vi "Traffic Light.vi"() -> ()   [LabVIEW 2013]
doc: "This VI is a simulation of traffic light.\nWere the traffic light controller provides for red,yellow and green light for every direction-\n-North Bound\n-South Bound\n-East Bound\n-West Bound\nAnd the second red, yellow and green list are provided for the left hand turn lane-\n-North Bound Left\n-South Bound Left\n-East Bound Left\n-West Bound Left\n\nThe period of time that light will be on is\n-Red: 4 sec\n-Yellow: 2 sec\n-Greeen: 4 sec\n\nThe left turn sequence eill be ON only when there will be the vehicle on the sensor."
uses:
  Controls/Traffic light.ctl
  Controls/Traffic_light_left.ctl
  Controls/States.ctl
  Controls/Sensor.ctl
panel:
  out "Enum":T1
  in  "North  Sensor":bool
  in  "Start":bool caption="stop"
  out "South Bound Left":T2
  out "South Bound":T3={"R"=TRUE, "Y"=FALSE, "G"=FALSE}
  out "West Bound Left":T2
  out "West Bound":T3={"R"=TRUE, "Y"=FALSE, "G"=FALSE}
  out "East Bound Left":T2
  out "East Bound":T3={"R"=TRUE, "Y"=FALSE, "G"=FALSE}
  in  "stop":bool
  in  "West Sensor":bool
  in  "East Sensor":bool
  in  "South Sensor":bool
  out "North Bound Left":T2
  out "North Bound":T3={"R"=TRUE, "Y"=FALSE, "G"=FALSE}
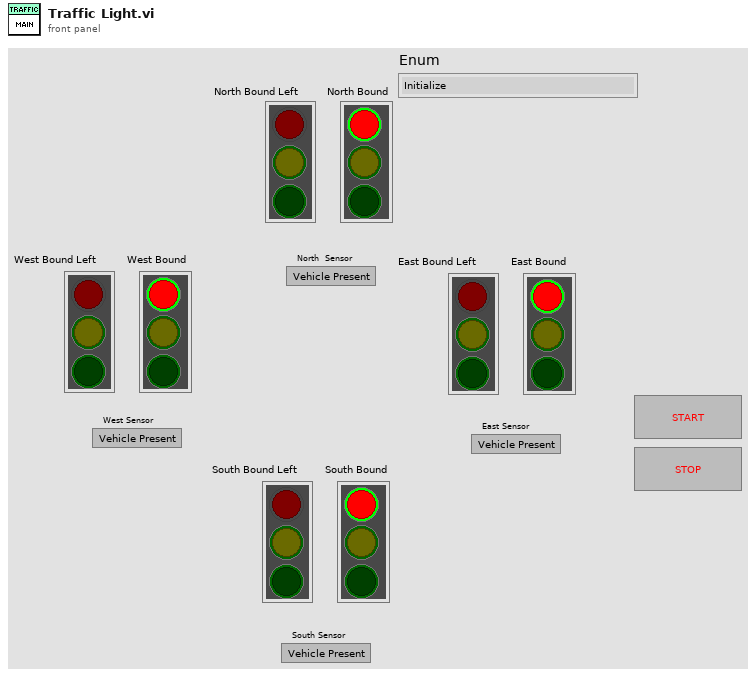
[diagram p1: front panel]
types:
  T1 = typedef "States.ctl" = enum16{"Initialize", "NS Green", "NS Yellow", "EW Green", "EW Yellow", "NS Left Green", "NS Left Yellow", "EW Left Green", "EW Left Yellow", "Stop"}
  T2 = typedef "Traffic_light_left.ctl" = cluster{"R":bool, "Y":bool, "G":bool}
  T3 = typedef "Traffic light.ctl" = cluster{"R":bool, "Y":bool, "G":bool}
  T4 = cluster{"North Bound":T3, "South Bound":T3, "East Bound":T3, "West Bound":T3, "North Bound Left":T2, "South Bound Left":T2, "East Bound Left":T2, "West Bound Left":T2}
  T5 = typedef "Sensor.ctl" = enum16{"Get", "Set"}
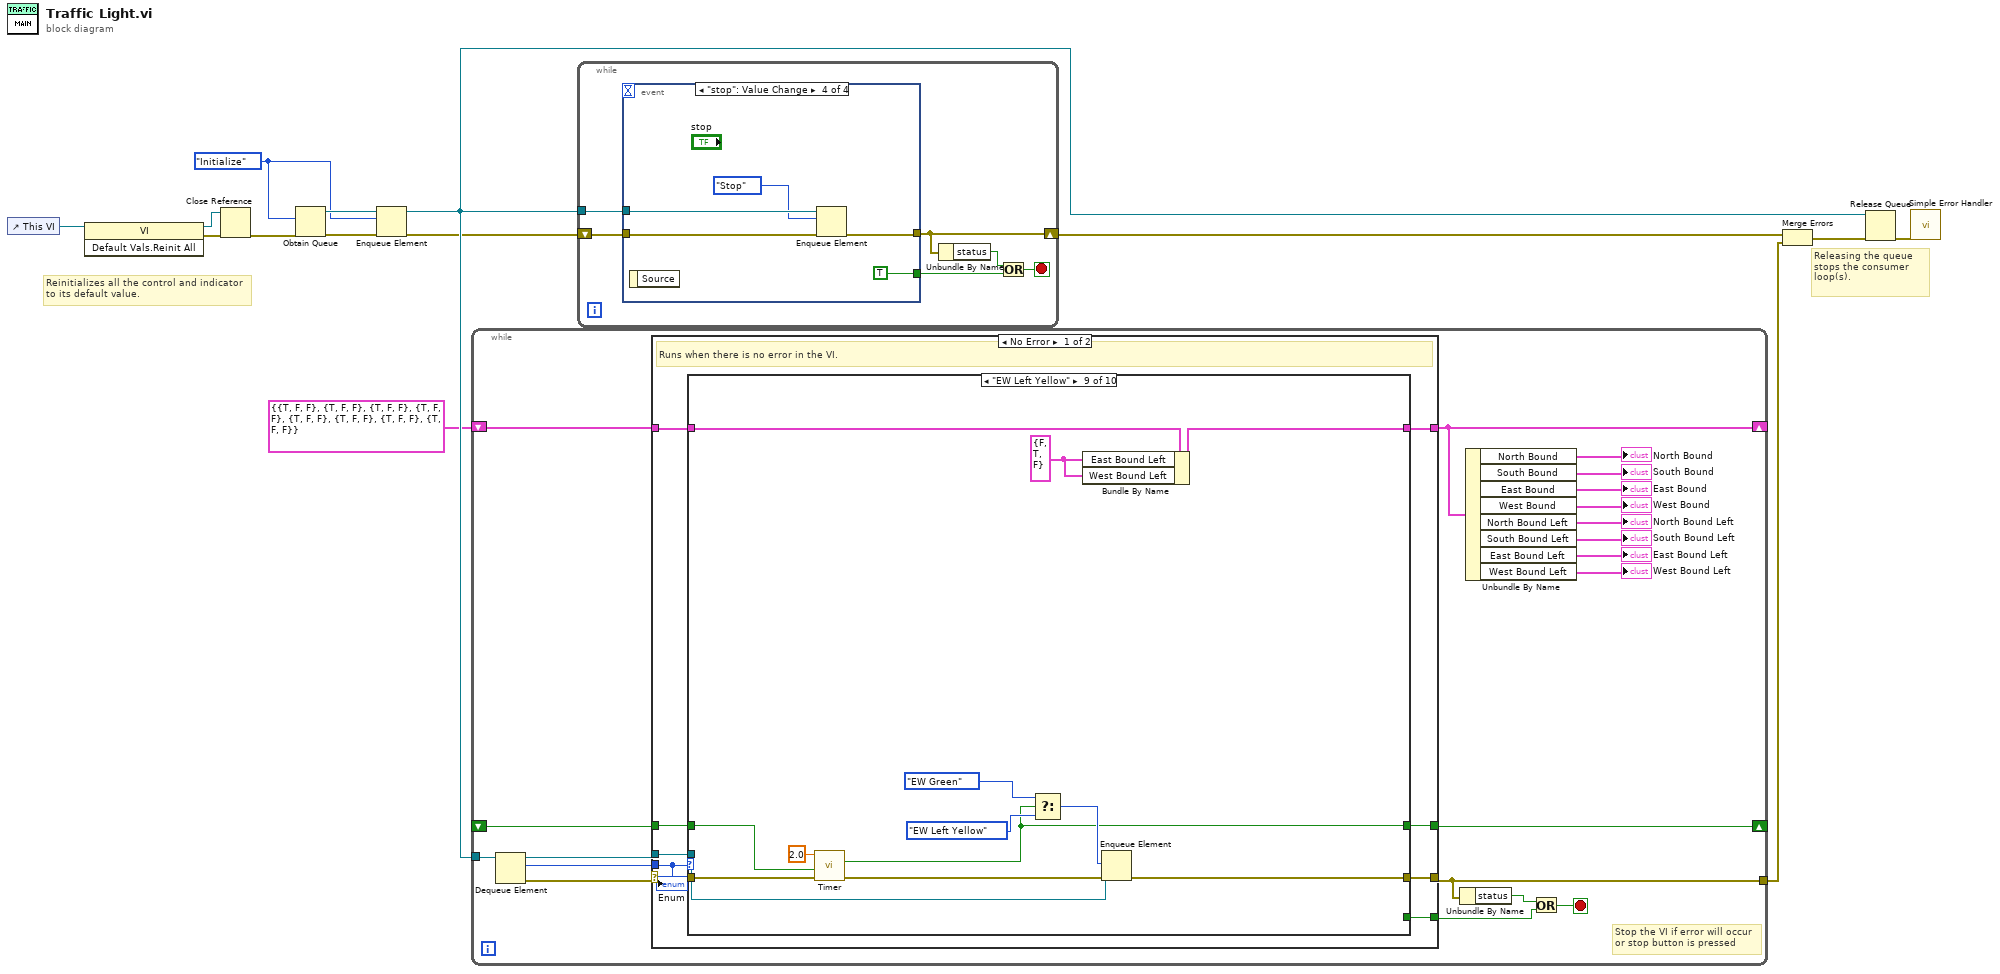
[diagram p0: block diagram]
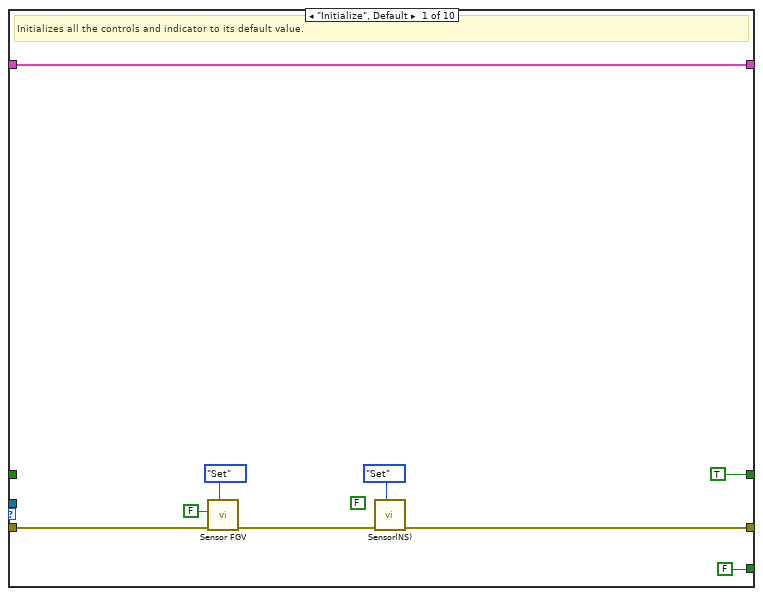
[diagram p2: hidden frame]
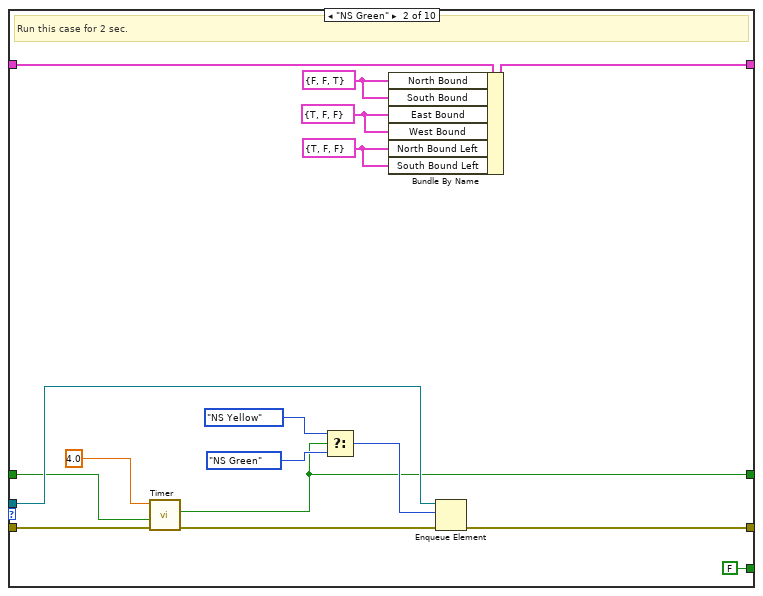
[diagram p3: hidden frame]
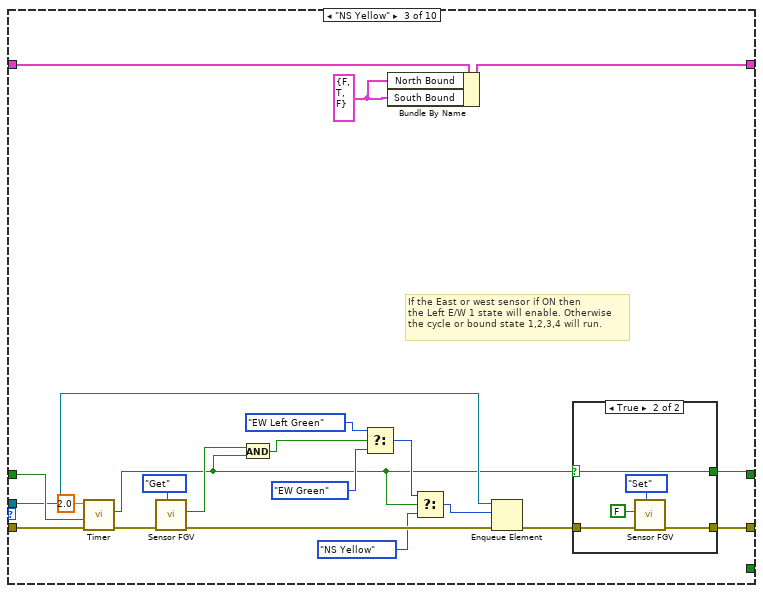
[diagram p4: hidden frame]
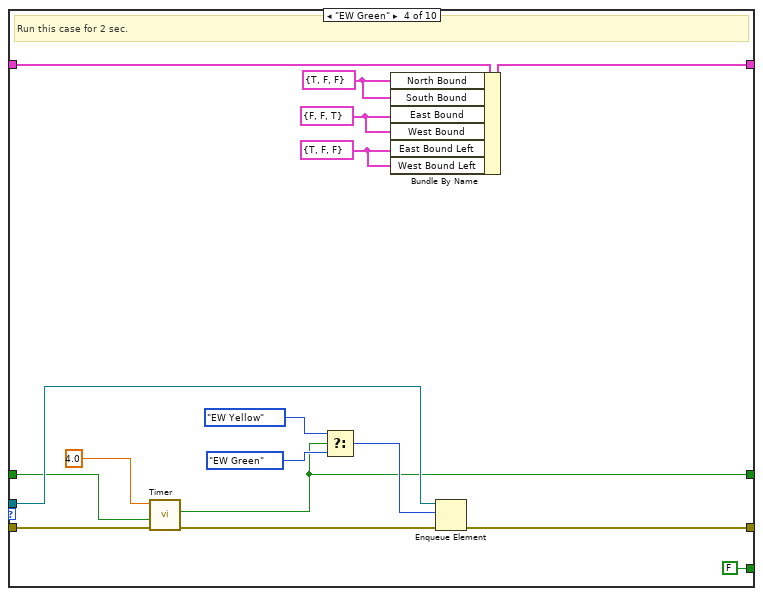
[diagram p6: hidden frame]
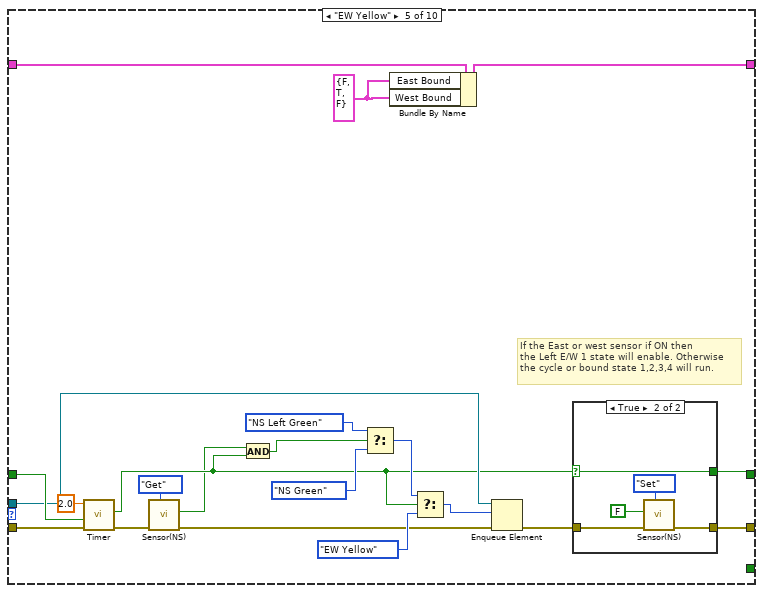
[diagram p7: hidden frame]
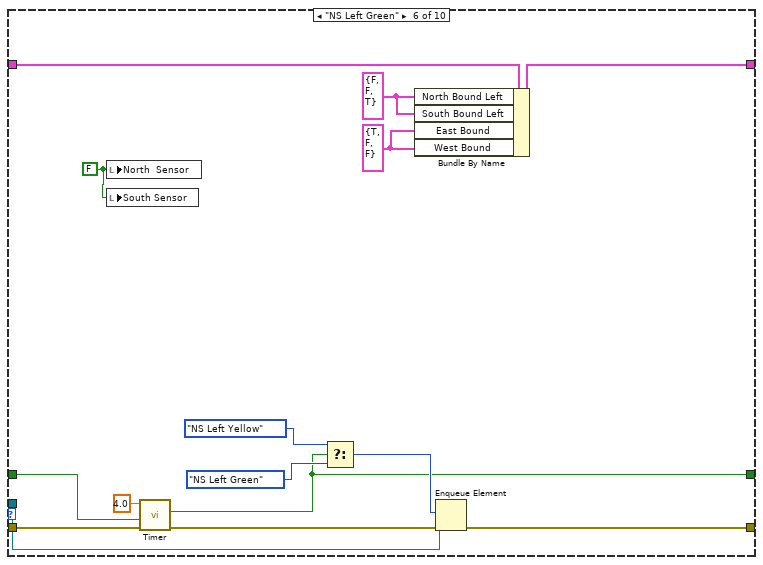
[diagram p9: hidden frame]
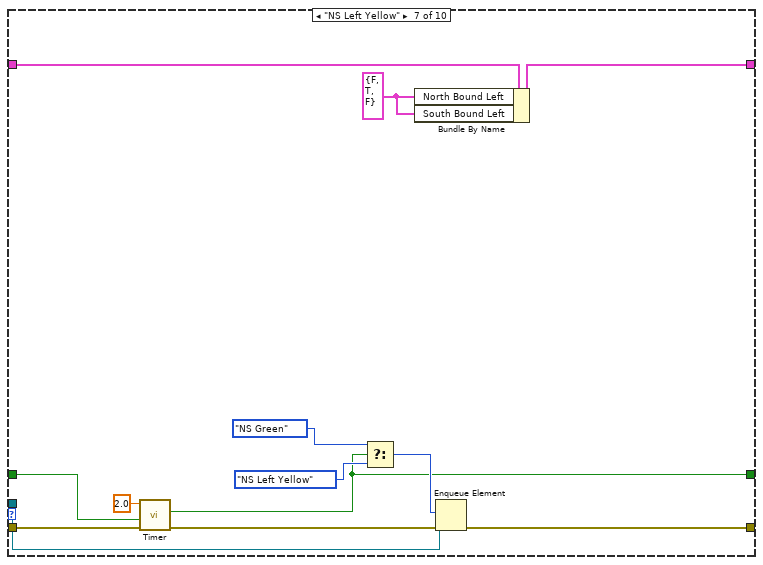
[diagram p10: hidden frame]
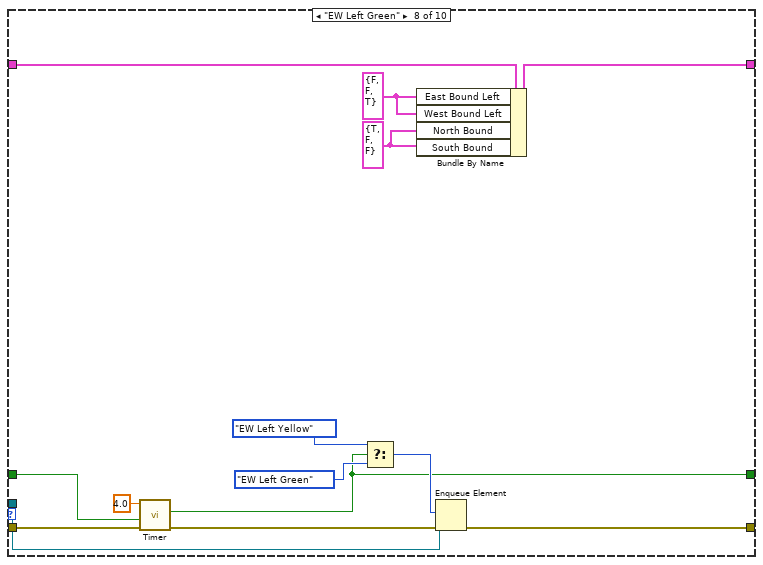
[diagram p11: hidden frame]
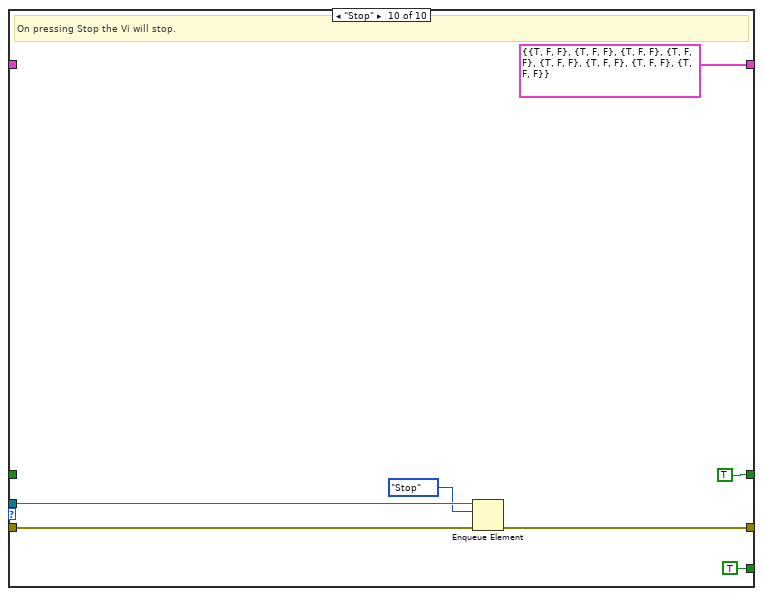
[diagram p12: hidden frame]
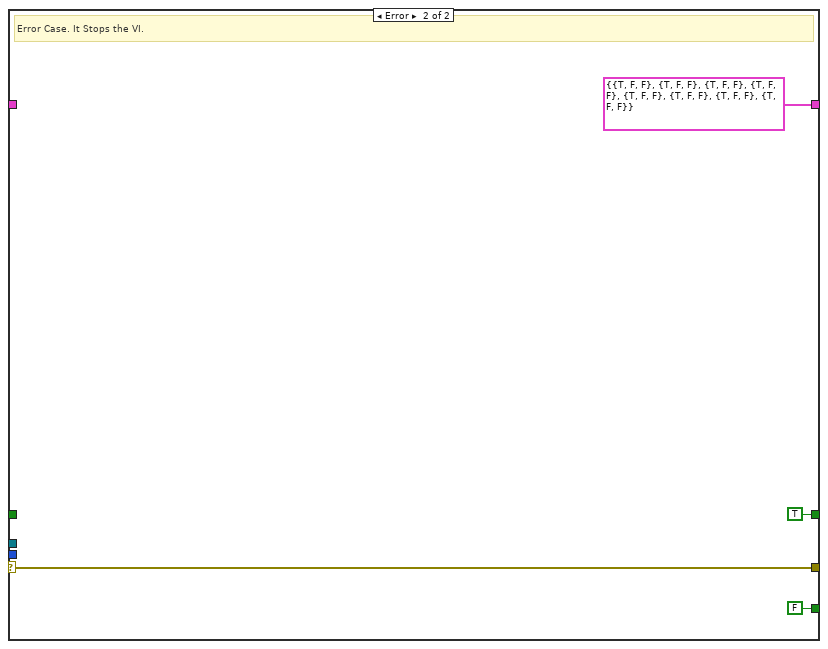
[diagram p13: hidden frame]
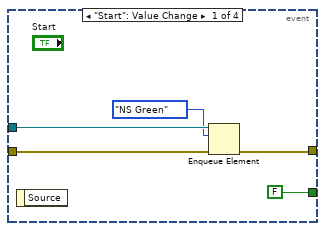
[diagram p14: hidden frame]
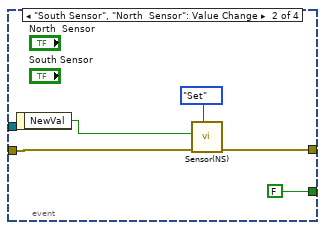
[diagram p15: hidden frame]
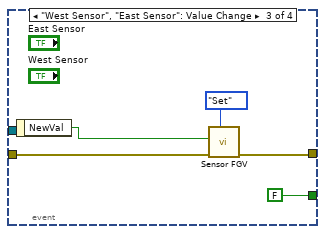
[diagram p16: hidden frame]
diagram:
  w10 = States."Initialize"
  # "Reinitializes all the control and indicator\nto its default value."
  # "Releasing the queue stops the consumer loop(s)."
  n1 = control-ref of="This VI"() -> (w9:refnum<vi>)
  n2 = invoke class="VI" method="Default Vals.Reinit All"(reference=w9) -> (reference out=w7:refnum<vi>, error out=w8:errorcluster)  [unwired: 2 in, 1 out]
  n3 = Close Reference(reference=w7, error in (no error)=w8) -> (error out=w6:errorcluster)
  n4 = Obtain Queue(element data type=w10, error in (no error)=w6) -> (queue out=w13:refnum<queue>, error out=w14:errorcluster)  [unwired: 3 in, 1 out]
  n5 = Enqueue Element(queue=w13, element=w10, error in (no error)=w14) -> (queue out=w12:refnum<queue>, error out=w11:errorcluster)  [unwired: 1 in, 1 out]
  n6 = while {
    tunnel: w12 -> [w34]
    shift-right: [w23] -> _
    shift-left: T4 {"North Bound"={"R"=TRUE, "Y"=FALSE, "G"=FALSE}, "South Bound"={"R"=TRUE, "Y"=FALSE, "G"=FALSE}, "East Bound"={"R"=TRUE, "Y"=FALSE, "G"=FALSE}, "West Bound"={"R"=TRUE, "Y"=FALSE, "G"=FALSE}, "North Bound Left"={"R"=TRUE, "Y"=FALSE, "G"=FALSE}, "South Bound Left"={"R"=TRUE, "Y"=FALSE, "G"=FALSE}, "East Bound Left"={"R"=TRUE, "Y"=FALSE, "G"=FALSE}, "West Bound Left"={"R"=TRUE, "Y"=FALSE, "G"=FALSE}} -> [w27]
    shift-right: [w25] -> _
    shift-left: _ -> [w26]
    tunnel: [w24] -> w4
    stop <- w30 stop-if-true
    # "Stop the VI if error will occur\nor stop button is pressed"
    n7 = Dequeue Element(queue=w34) -> (queue out=w31:refnum<queue>, element=w32:T1, error out=w33:errorcluster)  [unwired: 2 in, 1 out]
    n8 = case shown="No Error" w33 {
      selector: w33 -> [w42 w205]
      tunnel: w32 -> [w43 _]
      tunnel: w31 -> [w41 _]
      tunnel: [w40 w205] -> w24
      tunnel: [w39 FALSE] -> w28
      tunnel: w27 -> [w38 _]
      tunnel: [w37 T4 {"North Bound"={"R"=TRUE, "Y"=FALSE, "G"=FALSE}, "South Bound"={"R"=TRUE, "Y"=FALSE, "G"=FALSE}, "East Bound"={"R"=TRUE, "Y"=FALSE, "G"=FALSE}, "West Bound"={"R"=TRUE, "Y"=FALSE, "G"=FALSE}, "North Bound Left"={"R"=TRUE, "Y"=FALSE, "G"=FALSE}, "South Bound Left"={"R"=TRUE, "Y"=FALSE, "G"=FALSE}, "East Bound Left"={"R"=TRUE, "Y"=FALSE, "G"=FALSE}, "West Bound Left"={"R"=TRUE, "Y"=FALSE, "G"=FALSE}}] -> w23
      tunnel: w26 -> [w36 _]
      tunnel: [w35 TRUE ("Elapsed?")] -> w25
      frame No Error {
        # "Runs when there is no error in the VI."
        n9 = case shown="\"EW Left Yellow\"" w43 {
          tunnel: w42 -> [w49 w58 w81 w102 w127 w145 w159 w173 w186 w202]
          tunnel: w41 -> [_ w66 w85 w110 w130 w153 w166 w180 w193 w200]
          tunnel: [w46 w67 w73 w111 w121 w154 w167 w181 w194 w201] -> w40
          tunnel: [FALSE FALSE _ FALSE _ _ _ _ _ TRUE] -> w39
          tunnel: w38 -> [w51 w68 w89 w112 w133 w155 w168 w182 w195 _]
          tunnel: [w51 w56 w70 w100 w118 w143 w157 w171 w184 T4 {"North Bound"={"R"=TRUE, "Y"=FALSE, "G"=FALSE}, "South Bound"={"R"=TRUE, "Y"=FALSE, "G"=FALSE}, "East Bound"={"R"=TRUE, "Y"=FALSE, "G"=FALSE}, "West Bound"={"R"=TRUE, "Y"=FALSE, "G"=FALSE}, "North Bound Left"={"R"=TRUE, "Y"=FALSE, "G"=FALSE}, "South Bound Left"={"R"=TRUE, "Y"=FALSE, "G"=FALSE}, "East Bound Left"={"R"=TRUE, "Y"=FALSE, "G"=FALSE}, "West Bound Left"={"R"=TRUE, "Y"=FALSE, "G"=FALSE}}] -> w37
          tunnel: w36 -> [_ w65 w88 w109 w132 w152 w165 w179 w192 _]
          tunnel: [TRUE w61 w71 w105 w119 w148 w161 w175 w188 TRUE ("Elapsed?")] -> w35
          frame "Initialize", Default {
            (unwired) FALSE ("Boolean in")
            # "Initializes all the controls and indicator to its default value."
            n10 = call "Sensor FGV.vi"("Enum"=Sensor."Set", "error in (no error)"=w49, "Boolean in"=FALSE) -> ("error out"=w47:errorcluster)  [unwired: 7 in, 1 out]
            n11 = call "Sensor(NS) .vi"("Enum in"=Sensor."Set", "error in (no error)"=w47) -> ("error out"=w46:errorcluster)  [unwired: 8 in, 1 out]
          }
          frame "NS Green" {
            w53 = T2 {"R"=TRUE, "Y"=FALSE, "G"=FALSE} ("North Bound Left")
            w54 = T3 {"R"=TRUE, "Y"=FALSE, "G"=FALSE} ("East Bound")
            w55 = T3 {"R"=FALSE, "Y"=FALSE, "G"=TRUE} ("North Bound")
            # "Run this case for 2 sec."
            n12 = call "Timer.vi"("error in (no error)"=w58, "Reset"=w65, "Target"=4.0) -> ("error out"=w57:errorcluster, "Elapsed?"=w61:bool)  [unwired: 6 in, 1 out]
            n13 = Select(t=States."NS Yellow", s=w61, f=States."NS Green") -> (s? t:f=w62:T1)
            n14 = Bundle By Name(cluster=w68, "North Bound"=w55, "South Bound"=w55, "East Bound"=w54, "West Bound"=w54, "North Bound Left"=w53, "South Bound Left"=w53) -> (w56:T4)
            n15 = Enqueue Element(queue=w66, element=w62, error in (no error)=w57) -> (error out=w67:errorcluster)  [unwired: 1 in, 2 out]
          }
          frame "NS Yellow" {
            w69 = T3 {"R"=FALSE, "Y"=TRUE, "G"=FALSE} ("North Bound")
            # "If the East or west sensor if ON then \nthe Left E/W 1 state will enable. Otherwise\nthe cycle or bound state 1,2,3,4 will run."
            n16 = call "Timer.vi"("error in (no error)"=w81, "Reset"=w88, "Target"=2.0) -> ("error out"=w80:errorcluster, "Elapsed?"=w72:bool)  [unwired: 6 in, 1 out]
            n17 = call "Sensor FGV.vi"("Enum"=Sensor."Get", "error in (no error)"=w80) -> ("error out"=w86:errorcluster, "Boolean out"=w79:bool)  [unwired: 8 in]
            n18 = And(x=w79, y=w72) -> (x .and. y?=w78:bool)
            n19 = Select(t=States."EW Left Green", s=w78, f=States."EW Green") -> (s? t:f=w75:T1)
            n20 = Bundle By Name(cluster=w89, "North Bound"=w69, "South Bound"=w69) -> (w70:T4)
            n21 = Select(t=w75, s=w72, f=States."NS Yellow") -> (s? t:f=w82:T1)
            n22 = Enqueue Element(queue=w85, element=w82, error in (no error)=w86) -> (error out=w74:errorcluster)  [unwired: 1 in, 2 out]
            n23 = case shown="True" w72 {
              selector: w72 -> [w90 w94]
              tunnel: w74 -> [w91 w96]
              tunnel: [w91 w95] -> w73
              tunnel: [w90 w94] -> w71
              frame False {
              }
              frame True {
                n24 = call "Sensor FGV.vi"("Enum"=Sensor."Set", "error in (no error)"=w96, "Boolean in"=FALSE) -> ("error out"=w95:errorcluster)  [unwired: 7 in, 1 out]
              }
            }
          }
          frame "EW Green" {
            w97 = T2 {"R"=TRUE, "Y"=FALSE, "G"=FALSE} ("North Bound Left")
            w98 = T3 {"R"=FALSE, "Y"=FALSE, "G"=TRUE} ("East Bound")
            w99 = T3 {"R"=TRUE, "Y"=FALSE, "G"=FALSE} ("North Bound")
            # "Run this case for 2 sec."
            n25 = call "Timer.vi"("error in (no error)"=w102, "Reset"=w109, "Target"=4.0) -> ("error out"=w101:errorcluster, "Elapsed?"=w105:bool)  [unwired: 6 in, 1 out]
            n26 = Select(t=States."EW Yellow", s=w105, f=States."EW Green") -> (s? t:f=w106:T1)
            n27 = Bundle By Name(cluster=w112, "North Bound"=w99, "South Bound"=w99, "East Bound"=w98, "West Bound"=w98, "East Bound Left"=w97, "West Bound Left"=w97) -> (w100:T4)
            n28 = Enqueue Element(queue=w110, element=w106, error in (no error)=w101) -> (error out=w111:errorcluster)  [unwired: 1 in, 2 out]
          }
          frame "EW Yellow" {
            w117 = T3 {"R"=FALSE, "Y"=TRUE, "G"=FALSE} ("North Bound")
            # "If the East or west sensor if ON then \nthe Left E/W 1 state will enable. Otherwise\nthe cycle or bound state 1,2,3,4 will run."
            n29 = call "Timer.vi"("error in (no error)"=w127, "Reset"=w132, "Target"=2.0) -> ("error out"=w116:errorcluster, "Elapsed?"=w120:bool)  [unwired: 6 in, 1 out]
            n30 = call "Sensor(NS) .vi"("Enum in"=Sensor."Get", "error in (no error)"=w116) -> ("error out"=w115:errorcluster, "Boolean"=w114:bool)  [unwired: 8 in]
            n31 = And(x=w114, y=w120) -> (x .and. y?=w126:bool)
            n32 = Select(t=States."NS Left Green", s=w126, f=States."NS Green") -> (s? t:f=w123:T1)
            n33 = Bundle By Name(cluster=w133, "East Bound"=w117, "West Bound"=w117) -> (w118:T4)
            n34 = Select(t=w123, s=w120, f=States."EW Yellow") -> (s? t:f=w128:T1)
            n35 = Enqueue Element(queue=w130, element=w128, error in (no error)=w115) -> (error out=w122:errorcluster)  [unwired: 1 in, 2 out]
            n36 = case shown="True" w120 {
              selector: w120 -> [w134 w140]
              tunnel: w122 -> [w135 w138]
              tunnel: [w135 w137] -> w121
              tunnel: [w134 w140] -> w119
              frame False {
              }
              frame True {
                n37 = call "Sensor(NS) .vi"("Enum in"=Sensor."Set" ("Enum"), "error in (no error)"=w138, "Boolean in"=FALSE) -> ("error out"=w137:errorcluster)  [unwired: 7 in, 1 out]
              }
            }
          }
          frame "NS Left Green" {
            w141 = T2 {"R"=FALSE, "Y"=FALSE, "G"=TRUE} ("North Bound Left")
            w142 = T3 {"R"=TRUE, "Y"=FALSE, "G"=FALSE} ("East Bound")
            w146 = FALSE ("North  Sensor")
            n38 = local write "North  Sensor"(w146) -> ()
            n39 = local write "South Sensor"(w146) -> ()
            n40 = call "Timer.vi"("error in (no error)"=w145, "Reset"=w152, "Target"=4.0) -> ("error out"=w144:errorcluster, "Elapsed?"=w148:bool)  [unwired: 6 in, 1 out]
            n41 = Select(t=States."NS Left Yellow", s=w148, f=States."NS Left Green") -> (s? t:f=w149:T1)
            n42 = Bundle By Name(cluster=w155, "North Bound Left"=w141, "South Bound Left"=w141, "East Bound"=w142, "West Bound"=w142) -> (w143:T4)
            n43 = Enqueue Element(queue=w153, element=w149, error in (no error)=w144) -> (error out=w154:errorcluster)  [unwired: 1 in, 2 out]
          }
          frame "NS Left Yellow" {
            w156 = T2 {"R"=FALSE, "Y"=TRUE, "G"=FALSE} ("North Bound Left")
            n44 = call "Timer.vi"("error in (no error)"=w159, "Reset"=w165, "Target"=2.0) -> ("error out"=w158:errorcluster, "Elapsed?"=w161:bool)  [unwired: 6 in, 1 out]
            n45 = Select(t=States."NS Green", s=w161, f=States."NS Left Yellow") -> (s? t:f=w162:T1)
            n46 = Bundle By Name(cluster=w168, "North Bound Left"=w156, "South Bound Left"=w156) -> (w157:T4)
            n47 = Enqueue Element(queue=w166, element=w162, error in (no error)=w158) -> (error out=w167:errorcluster)  [unwired: 1 in, 2 out]
          }
          frame "EW Left Green" {
            w169 = T3 {"R"=TRUE, "Y"=FALSE, "G"=FALSE} ("North Bound")
            w170 = T2 {"R"=FALSE, "Y"=FALSE, "G"=TRUE} ("North Bound Left")
            n48 = call "Timer.vi"("error in (no error)"=w173, "Reset"=w179, "Target"=4.0) -> ("error out"=w172:errorcluster, "Elapsed?"=w175:bool)  [unwired: 6 in, 1 out]
            n49 = Select(t=States."EW Left Yellow", s=w175, f=States."EW Left Green") -> (s? t:f=w176:T1)
            n50 = Bundle By Name(cluster=w182, "East Bound Left"=w170, "West Bound Left"=w170, "North Bound"=w169, "South Bound"=w169) -> (w171:T4)
            n51 = Enqueue Element(queue=w180, element=w176, error in (no error)=w172) -> (error out=w181:errorcluster)  [unwired: 1 in, 2 out]
          }
          frame "EW Left Yellow" {
            w183 = T2 {"R"=FALSE, "Y"=TRUE, "G"=FALSE} ("North Bound Left")
            n52 = call "Timer.vi"("error in (no error)"=w186, "Reset"=w192, "Target"=2.0) -> ("error out"=w185:errorcluster, "Elapsed?"=w188:bool)  [unwired: 6 in, 1 out]
            n53 = Select(t=States."EW Green", s=w188, f=States."EW Left Yellow") -> (s? t:f=w189:T1)
            n54 = Bundle By Name(cluster=w195, "East Bound Left"=w183, "West Bound Left"=w183) -> (w184:T4)
            n55 = Enqueue Element(queue=w193, element=w189, error in (no error)=w185) -> (error out=w194:errorcluster)  [unwired: 1 in, 2 out]
          }
          frame "Stop" {
            # "On pressing Stop the Vi will stop."
            n56 = Enqueue Element(queue=w200, element=States."Stop", error in (no error)=w202) -> (error out=w201:errorcluster)  [unwired: 1 in, 2 out]
          }
        }
        "Enum" <- w43
      }
      frame Error {
        # "Error Case. It Stops the VI."
      }
    }
    n57 = Unbundle By Name(w24) -> ("status"=w29:bool)
    n58 = Unbundle By Name(w23) -> ("North Bound"=→"North Bound":T3, "South Bound"=→"South Bound":T3, "East Bound"=→"East Bound":T3, "West Bound"=→"West Bound":T3, "North Bound Left"=→"North Bound Left":T2, "South Bound Left"=→"South Bound Left":T2, "East Bound Left"=→"East Bound Left":T2, "West Bound Left"=→"West Bound Left":T2)
    n59 = Or(x=w29, y=w28) -> (x .or. y?=w30:bool)
  }
  n60 = while {
    shift-right: [w209] -> w5
    shift-left: w11 -> [w211]
    tunnel: w12 -> [w212]
    stop <- w210 stop-if-true
    n61 = event shown="[3] \"stop\": Value Change" {
      selector: _ -> [_ _ _ _]
      dyn-events: _ -> [_ _ _ _]
      timeout: _ -> [_ _ _ _]
      tunnel: w212 -> [w215 _ _ w230]
      tunnel: w211 -> [w217 w221 w226 w232]
      tunnel: [w216 w220 w225 w231] -> w209
      tunnel: [FALSE FALSE FALSE TRUE] -> w207
      event "Start": Value Change {
        n62 = event-data() -> ()  [unwired: 1 in, 1 out]
        n63 = Enqueue Element(queue=w215, element=States."NS Green", error in (no error)=w217) -> (error out=w216:errorcluster)  [unwired: 1 in, 2 out]
      }
      event "South Sensor", "North  Sensor": Value Change {
        n64 = event-data() -> ("NewVal"=w218:bool)  [unwired: 1 in]
        n65 = call "Sensor(NS) .vi"("Enum in"=Sensor."Set", "error in (no error)"=w221, "Boolean in"=w218) -> ("error out"=w220:errorcluster)  [unwired: 7 in, 1 out]
      }
      event "West Sensor", "East Sensor": Value Change {
        n66 = event-data() -> ("NewVal"=w223:bool)  [unwired: 1 in]
        n67 = call "Sensor FGV.vi"("Enum"=Sensor."Set", "error in (no error)"=w226, "Boolean in"=w223) -> ("error out"=w225:errorcluster)  [unwired: 7 in, 1 out]
      }
      event "stop": Value Change {
        n68 = event-data() -> ()  [unwired: 1 in, 1 out]
        n69 = Enqueue Element(queue=w230, element=States."Stop", error in (no error)=w232) -> (error out=w231:errorcluster)  [unwired: 1 in, 2 out]
      }
    }
    n70 = Unbundle By Name(w209) -> ("status"=w208:bool)
    n71 = Or(x=w208, y=w207) -> (x .or. y?=w210:bool)
  }
  n72 = Merge Errors(w5, w4) -> (w3:errorcluster)
  n73 = Release Queue(queue=w12, error in (no error)=w3) -> (error out=w2:errorcluster)  [unwired: 1 in, 2 out]
  n74 = call <vilib>:"Simple Error Handler.vi"("error in (no error)"=w2) -> ()  [unwired: 4 in, 5 out]
